vi "Approach.vi"(7 "Computer called (T/F)":bool) -> ()   [LabVIEW 2023]
uses:
  Sub_Vi/TypeDefsControls/Zposition.ctl
  Sub_Vi/TypeDefsControls/Piezo Velocity.ctl
  Sub_Vi/TypeDefsControls/Voltage.ctl
  Sub_Vi/TypeDefsControls/Xposition.ctl
  Sub_Vi/TypeDefsControls/Yposition.ctl
  Sub_Vi/TypeDefsControls/Feedback Type.ctl
  Sub_Vi/TypeDefs/WayPointCluster.ctl
  Sub_Vi/TypeDefs/Settings.ctl
  Sub_Vi/TypeDefs/ChangeOnFly.ctl
  Sub_Vi/TypeDefs/Display.ctl
  Settings.vi
panel:
  out "Current 5":cluster{"Y":dbl[], "Y":dbl[]}[](graph)
  out "Current 4":cluster{"Y":dbl[], "Y":dbl[]}[](graph)
  out "Lock In Phase":dbl[](graph)
  out "Lock In Amplitude":dbl[](graph)
  in  "Start scan Button":bool
  in  "Retract after approach over":bool=TRUE
  in  "Display Cluster":T1
  in  "ChangeonFly":T2
  in  "SettingsCluster":T3={"Sample Rate (us)"=1, "Samples Per Data Point (int, power of 2)"=1000, "DistanceToBulk (um)"=-1.0, "HoldTimeScaler"=1, "SaveData"=TRUE, "DistanceToBulk (um) 2"=-1.0, "DistanceToBulk (um) 3"=-1.0}
  in  "WayPointCluster":T4
  in  "Feedback Type":T5=enum."Current 1"
  in  "Tab Control":enum32{"Current-Distance", "Current-Time"}(tab)
  out "Current 1":cluster{"Y":dbl[], "Y":dbl[]}[](graph)
  out "Current 2":cluster{"Y":dbl[], "Y":dbl[]}[](graph)
  out "Current 3":cluster{"Y":dbl[], "Y":dbl[]}[](graph)
  out "Current 1":dbl[](graph)
  out "Current 2":dbl[](graph)
  out "Current 3":dbl[](graph)
  in  "Feedback Threshold (A)":dbl=1e-13 min=-360.0 max=360.0
  in  "Greater Than":bool=TRUE
  in  "Set X":bool
  in  "Set Y":bool
  in  "Y (µm)":T6=50.0 min=0.0 max=100000.0
  in  "X (µm)":T7=50.0 min=0.0 max=100000.0
  in  "Approach Voltage (V)":T8=0.35 min=-10.0 max=10.0
  in  "Approach Rate (µm/s)":T9=0.1 min=0.0
  in  "End Extension (µm)":T10 min=0.0 max=100000.0
  in  "Start Extention (µm)":T10=150.0 min=0.0 max=100000.0
  in  "stop 2":bool
  in  "Pause":bool
  # "Settings"
  # "Pause at"
  # "Advanced Settings"
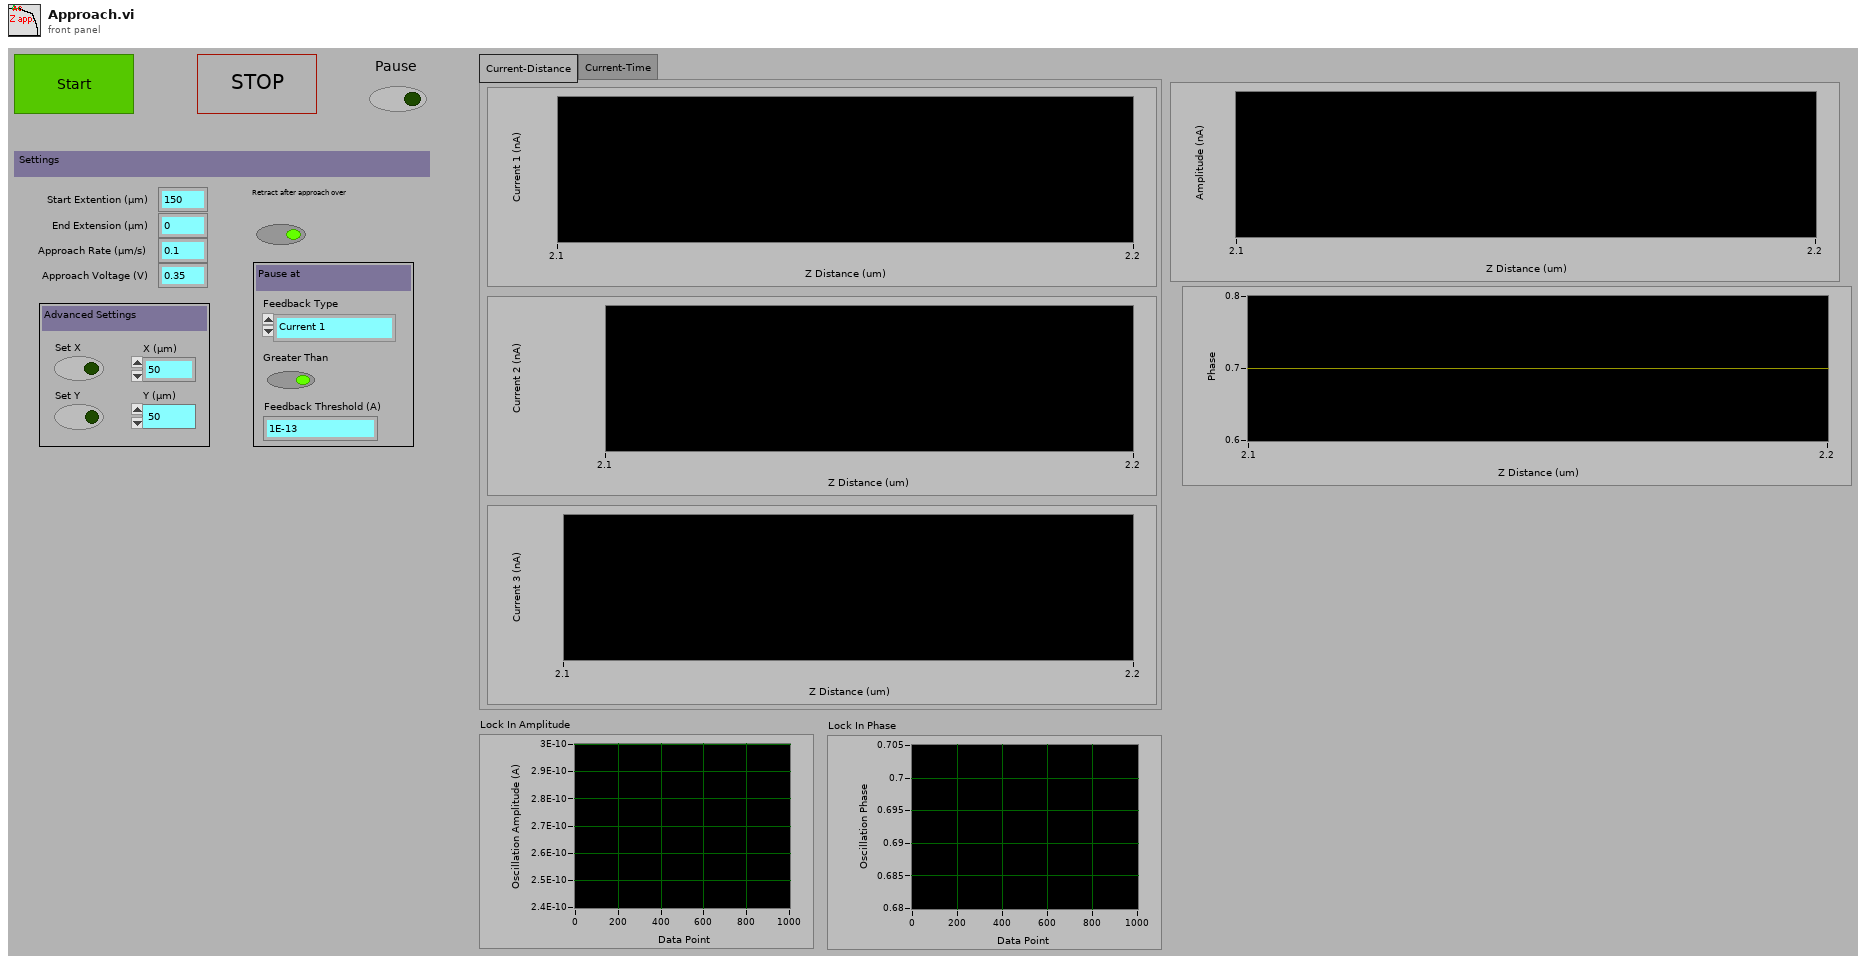
[diagram p1: front panel]
types:
  T1 = typedef "Display.ctl" = cluster{"X":refnum<vi>, "Y":refnum<vi>, "Z":refnum<vi>, "Amp":refnum<vi>, "Phase":refnum<vi>, "t vs Z":refnum<vi>, "t vs C1":refnum<vi>, "t vs C2":refnum<vi>, "t vs C3":refnum<vi>, "t vs Amp":refnum<vi>, "t vs Phase":refnum<vi>, "t vs X":refnum<vi>, "t vs Y":refnum<vi>, "Z vs C1":refnum<vi>, "Z vs C2":refnum<vi>, "Z vs C3":refnum<vi>, "V vs C1":refnum<vi>, "V vs C2":refnum<vi>, "V vs C3":refnum<vi>, "X/Y/Z F":refnum<vi>, "X/Y/Z R":refnum<vi>, "X/Y/C1 F":refnum<vi>, "X/Y/C1 R":refnum<vi>, "X/Y/C2 F":refnum<vi>, "X/Y/C2 R":refnum<vi>, "X/Y/C3 F":refnum<vi>, "X/Y/C3 R":refnum<vi>, "NumberOfLines":u16, "um Per Pixel":dbl, "um Per Line":dbl, "X Center":dbl, "Hop X/Y/Z":refnum<vi>, "Hop X/Y/C1":refnum<vi>, "Hop X/Y/C2":refnum<vi>, "Hop X/Y/C3":refnum<vi>, "X Width":dbl, "Y Width":dbl, "Hopping Distance":dbl, "V2 vs C1":refnum<vi>, "V vs Phase":refnum<vi>, "Y Center":dbl, "Number of Pixels":dbl, "V2 vs C2":refnum<vi>, "V2 vs C3":refnum<vi>, "V vs y":refnum<vi>, "V2 vs y":refnum<vi>, "Z vs Amp":refnum<vi>, "Z vs Phase":refnum<vi>}
  T2 = typedef "ChangeOnFly.ctl" = cluster{"Stop (boolean)":refnum<vi>, "Pause (boolean)":refnum<vi>, "EndCurrentLine (boolean)":refnum<vi>, "max movement per update step (Interger, nm)":refnum<vi>, "P (float, arb)":refnum<vi>, "Feedback set point (double, Amps)":refnum<vi>, "Voltage (double, V)":refnum<vi>, "Feedback set point 2 (double, Amps)":refnum<vi>, "Stop on Greater Than 2? (boolean)":refnum<vi>, "Stop on Greater Than? (boolean)":refnum<vi>, "Voltage 2 (double, V)":refnum<vi>, "Feedback Type (enum)":refnum<vi>, "Feedback Type 2 (enum)":refnum<vi>}
  T3 = typedef "Settings.ctl" = cluster{"Sample Rate (us)":u32, "Samples Per Data Point (int, power of 2)":i16, "DistanceToBulk (um)":dbl, "HoldTimeScaler":u64, "SaveData":bool, "DistanceToBulk (um) 2":dbl, "DistanceToBulk (um) 3":dbl}
  T4 = typedef "WayPointCluster.ctl" = cluster{"X (um)":dbl[], "Y (um)":dbl[], "Z (um)":dbl[], "V (V)":dbl[], "X Velocity (um s-1)":dbl[], "Y Velocity (um s-1)":dbl[], "Z Velocity (um s-1)":dbl[], "V Velocity (V s-1)":dbl[], "FeedBack Type (enum)":u16[], "Move X (boolean)":bool[], "Move Y (boolean)":bool[], "Move Z (boolean)":bool[], "Move V (boolean)":bool[], "Jump V (boolean)":bool[], "Hold (boolean)":bool[], "Hold Time":u32[], "V2 (V)":dbl[], "Move V2":bool[], "V2 Velocity (V s-1)":dbl[], "Jump V2 (boolean)":bool[], "Update z Position delta (ms)":i16[], "Hold Feedback1":bool[], "Move Z PicoMotor":bool[], " Z PicoMotor Direction":bool[], "DIO0":bool[]}
  T5 = typedef "Feedback Type.ctl" = enum16{"AC Magnitude", "Current 1", "Current 2", "Phase"}
  T6 = typedef "Yposition.ctl" = dbl
  T7 = typedef "Xposition.ctl" = dbl
  T8 = typedef "Voltage.ctl" = dbl
  T9 = typedef "Piezo Velocity.ctl" = dbl
  T10 = typedef "Zposition.ctl" = dbl
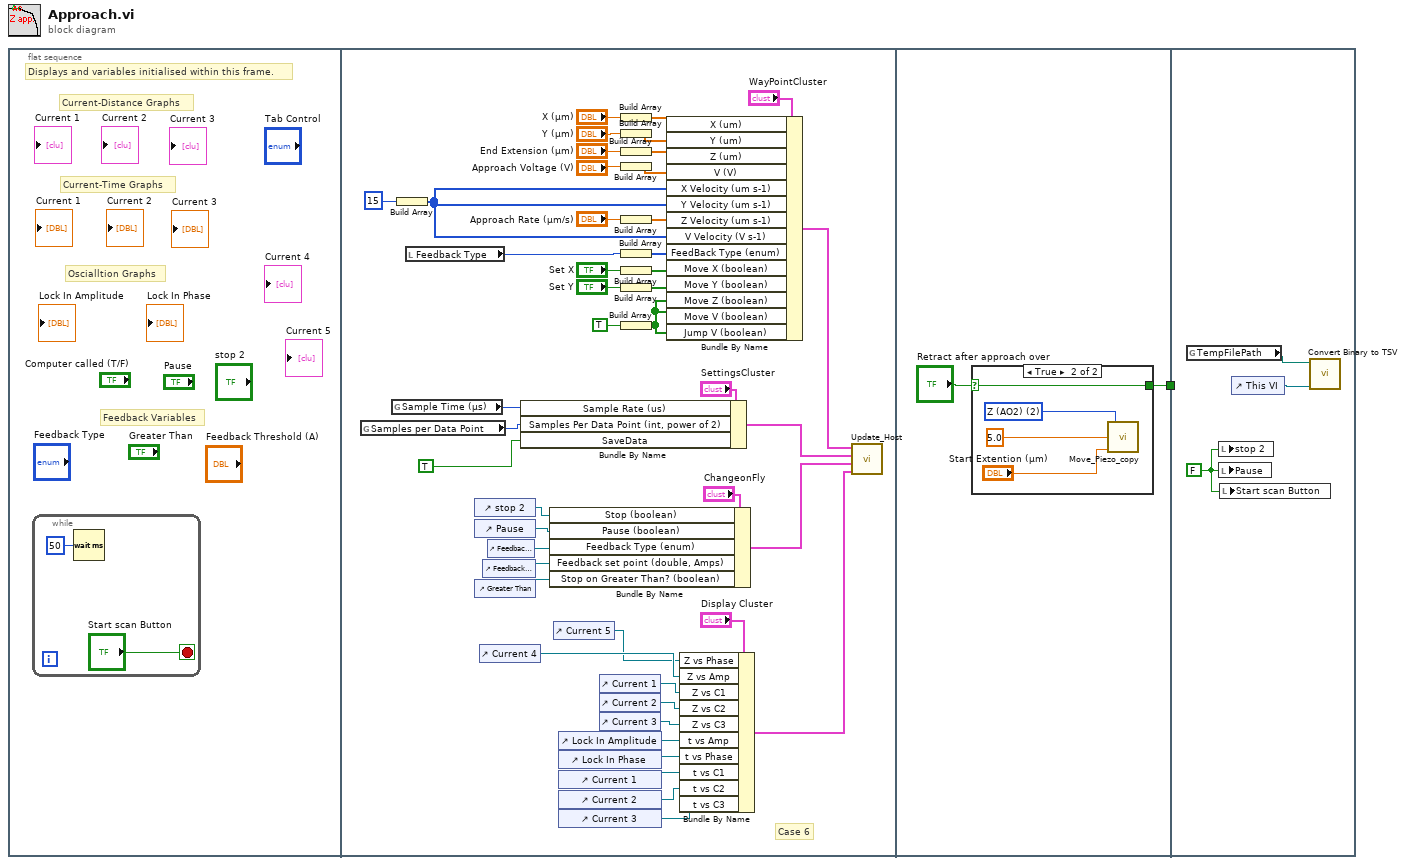
[diagram p0: block diagram]
diagram:
  n1 = flat-sequence {
    tunnel: [w50] -> w1
    tunnel: w1 -> [_]
    frame #0 {
      # "Feedback Variables"
      # "Oscialltion Graphs"
      # "Current-Time Graphs"
      # "Current-Distance Graphs"
      # "Displays and variables initialised within this frame."
      n2 = while {
        stop <- "Start scan Button" stop-if-true
        n3 = Wait (ms)(milliseconds to wait=u32 50) -> ()  [unwired: 1 out]
      }
    }
    frame #1 {
      # "Case 6"
      n4 = global read "Settings.vi" "Samples per Data Point"() -> (w26:u16)
      n5 = global read "Settings.vi" "Sample Time (µs)"() -> (w27:u32)
      n6 = Build Array(15) -> (w49:i32[])
      n7 = local read "Feedback Type"() -> (w4:T5)
      n8 = control-ref of="stop 2"() -> (w20:refnum<vi>)
      n9 = control-ref of="Pause"() -> (w38:refnum<vi>)
      n10 = control-ref of="Greater Than"() -> (w25:refnum<vi>)
      n11 = control-ref of="Current 4"() -> (w7:refnum<vi>)
      n12 = control-ref of="Feedback Threshold (A)"() -> (w39:refnum<vi>)
      n13 = control-ref of="Feedback Type"() -> (w24:refnum<vi>)
      n14 = Bundle By Name(cluster="SettingsCluster", "Sample Rate (us)"=w27, "Samples Per Data Point (int, power of 2)"=w26, "SaveData"=TRUE) -> (w10:T3)
      n15 = Bundle By Name(cluster="ChangeonFly", "Stop (boolean)"=w20, "Pause (boolean)"=w38, "Feedback Type (enum)"=w24, "Feedback set point (double, Amps)"=w39, "Stop on Greater Than? (boolean)"=w25) -> (w9:T2)
      n16 = control-ref of="Current 5"() -> (w6:refnum<vi>)
      n17 = control-ref of="Lock In Amplitude"() -> (w8:refnum<vi>)
      n18 = control-ref of="Lock In Phase"() -> (w36:refnum<vi>)
      n19 = control-ref of="Current 1"() -> (w17:refnum<vi>)
      n20 = control-ref of="Current 2"() -> (w21:refnum<vi>)
      n21 = control-ref of="Current 3"() -> (w35:refnum<vi>)
      n22 = control-ref of="Current 1"() -> (w43:refnum<vi>)
      n23 = control-ref of="Current 2"() -> (w18:refnum<vi>)
      n24 = control-ref of="Current 3"() -> (w19:refnum<vi>)
      n25 = Build Array("X (µm)") -> (w48:T7[])
      n26 = Build Array("Y (µm)") -> (w47:T6[])
      n27 = Build Array("End Extension (µm)") -> (w45:T10[])
      n28 = Build Array("Approach Voltage (V)") -> (w46:T8[])
      n29 = Build Array("Approach Rate (µm/s)") -> (w44:T9[])
      n30 = Build Array(w4) -> (w42:T5[])
      n31 = Build Array("Set X") -> (w41:bool[])
      n32 = Build Array("Set Y") -> (w40:bool[])
      n33 = Build Array(TRUE ("Save Data")) -> (w23:bool[])
      n34 = Bundle By Name(cluster="WayPointCluster", "X (um)"=w48, "Y (um)"=w47, "Z (um)"=w45, "V (V)"=w46, "X Velocity (um s-1)"=w49, "Y Velocity (um s-1)"=w49, "Z Velocity (um s-1)"=w44, "V Velocity (V s-1)"=w49, "FeedBack Type (enum)"=w42, "Move X (boolean)"=w41, "Move Y (boolean)"=w40, "Move Z (boolean)"=w23, "Move V (boolean)"=w23, "Jump V (boolean)"=w23) -> (w11:T4)
      n35 = Bundle By Name(cluster="Display Cluster", "Z vs Phase"=w6, "Z vs Amp"=w7, "Z vs C1"=w43, "Z vs C2"=w18, "Z vs C3"=w19, "t vs Amp"=w8, "t vs Phase"=w36, "t vs C1"=w17, "t vs C2"=w21, "t vs C3"=w35) -> (w22:T1)
      n36 = call "Update_Host.vi"("Display Cluster"=w22, "ChangeonFly"=w9, "SettingsCluster"=w10, "WayPointCluster"=w11) -> ()  [unwired: 6 in]
    }
    frame #2 {
      n37 = case shown="True" "Retract after approach over" {
        selector: "Retract after approach over" -> [w52 w55]
        tunnel: [w52 w55] -> w50
        frame False {
        }
        frame True {
          w56 = u16 2 items=["X (AO0)", "Y (AO1)", "Z (AO2)", "V (AO3)", "V2 (AO4)"] ("Piezo")
          n38 = call "Move_Piezo_copy.vi"("Piezo"=w56, "Movement Speed (µm/s)"=5.0 ("Scan Rate (um/s)"), "Position (µm) (or V)"="Start Extention (µm)") -> ()  [unwired: 13 in]
        }
      }
    }
    frame #3 {
      w58 = FALSE ("stop recording")
      n39 = global read "Settings.vi" "TempFilePath"() -> (w57:path)
      n40 = local write "stop 2"(w58) -> ()
      n41 = local write "Pause"(w58) -> ()
      n42 = local write "Start scan Button"(w58) -> ()
      n43 = control-ref of="This VI"() -> (w59:refnum<vi>)
      n44 = call "Convert Binary to TSV.vi"("This VI"=w59, "TDMS DataFile Name"=w57) -> ()  [unwired: 10 in]
    }
  }
